vi "hdt_main_averageChannels.vi"(8 "outSteamSelect":u8(ring) items=["PID/ORT", "SICM"], 10 "hdt.p.averageEnabled":bool=TRUE, 11 "enableOutput":bool) -> (0 "debugStream":T1)   [LabVIEW 2016]
uses:
  <vilib>/rvi/Emulation/niFpgaEmulationIsFPGAContextNoSignature.vi
  <vilib>/rvi/Emulation/niFpgaSctlEmulationGetInTimedLoop.vi
  <vilib>/rvi/errors/niFpgaSetErrorForExecOnDevCompSimple.vi
  <vilib>/rvi/eio/common/nirviEmuReportErrorAndStop.vi
  <vilib>/rvi/DataTransferAndStorage/Container/Common/niFpgaContainerGetUniqueNameForEmu.vi
  <vilib>/rvi/FIFO/Fifo_Resource/nirvififoEmulationSetSize.vi
  <vilib>/rvi/FIFO/Fifo_Resource/nirviFifoEmulationQueueMgr.vi
  <instcachedir>/0/nirviFifoEmulationQueueMgr_E5CAEC123FF24DC58D834DCA3CDAA9B5.lvgen/nirviFifoEmulationQueueMgr_E5CAEC123FF24DC58D834DCA3CDAA9B5_010.vi
  <vilib>/Utility/error.llb/Clear Errors.vi
  <vilib>/rvi/FIFO/Fifo_Resource/nirvififoEmulationCreateLock.vi
  <vilib>/rvi/Emulation/niFpgaProcessEmulError.vi
  <vilib>/rvi/FIFO/Fifo_Resource/nirvififoEmulationObtainLock.vi
  <vilib>/rvi/FIFO/Fifo_Resource/nirvififoEmulationReleaseLock.vi
  <vilib>/rvi/occurrence/nirviWaitOnOccurrenceBase.vi
  <vilib>/rvi/errors/nirviReportUnexpectedCaseInternalError.vi
  <vilib>/rvi/errors/nirviReportUnexpectedCaseInternalError (U32).vi
  <instcachedir>/0/nirviFifoEmulationQueueMgr_E5CAEC123FF24DC58D834DCA3CDAA9B5.lvgen/nirviFifoEmulationQueueMgr_E5CAEC123FF24DC58D834DCA3CDAA9B5_009.vi
  <vilib>/rvi/FIFO/Fifo_Resource/nirvififoEmulationDetermineInputValidOut.vi
  <vilib>/rvi/DataTransferAndStorage/Container/XNode/niFpgaContainer.xnode
  <vilib>/rvi/FIFO/Fifo_Resource/nirvififoEmulationRead.vi
  <vilib>/rvi/FXPMathLib/FxpInterpret/XNode/nifxpmath_Interpret.xnode
  <vilib>/rvi/FIFO/Fifo_Resource/nirvififoEmulationWrite.vi
  <vilib>/eio/EIONode/EIONode.xnode
  <vilib>/rvi/eio/common/nirviEmuTemplateMethod_errors.vi
  <vilib>/rvi/DataTransferAndStorage/Register/Emulation/niFpgaRegisterEmulation.vi
types:
  T1 = cluster{"ch2":fxp<+/-,22,1>, "ch3":fxp<+/-,22,1>}
  T2 = cluster{"Element":fxp<+/-,22,1>, "Element":fxp<+/-,22,1>}
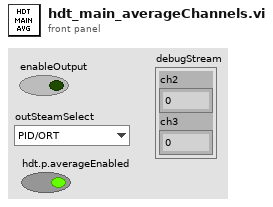
[diagram p1: front panel]
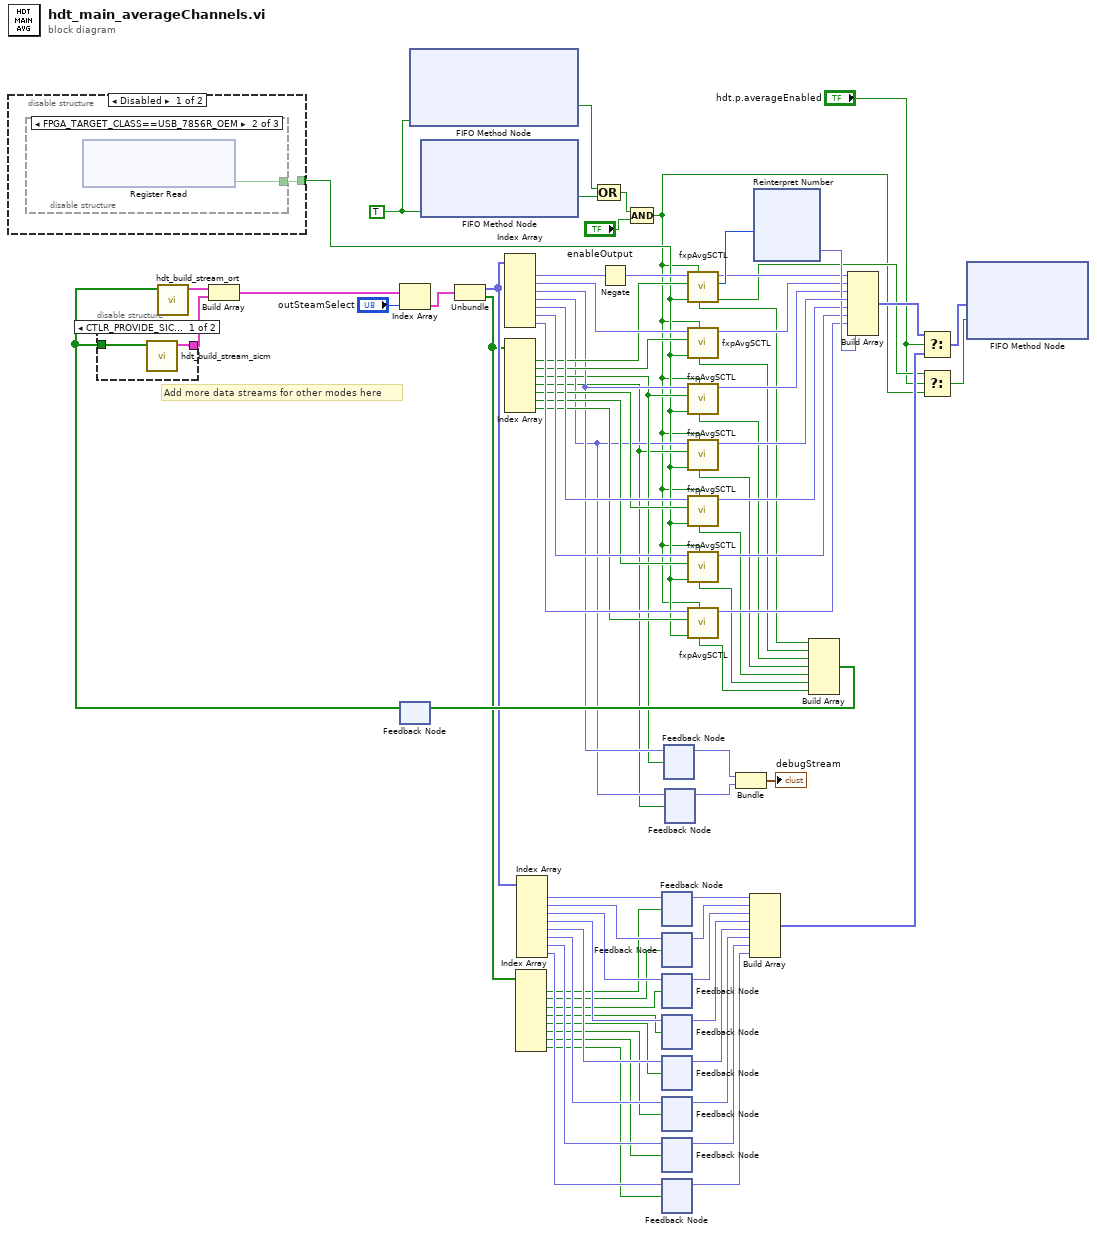
[diagram p0: block diagram]
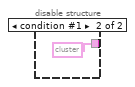
[diagram p2: hidden frame]
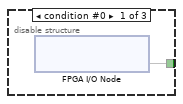
[diagram p3: hidden frame]
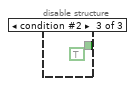
[diagram p4: hidden frame]
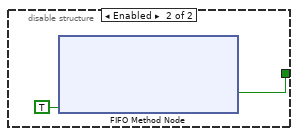
[diagram p5: hidden frame]
diagram:
  w43 = TRUE ("Ready for Output")
  # "Add more data streams for other modes here"
  n1 = disable-structure shown="Disabled" {
    disable-tunnel: [w81 w86] -> w34
    frame Disabled {
      n2 = disable-structure shown="FPGA_TARGET_CLASS==USB_7856R_OEM" {
        disable-tunnel: [w82 w83 TRUE ("outputEnable")] -> w81
        frame condition #0 {
          n3 = xnode "FPGA I/O Node"() -> ("outputEnable"=w82)  [unwired: 1 in, 1 out]
        }
        frame condition #1 (active) {
          n4 = xnode ("Register Read")() -> ("Data"=w83:bool)  [unwired: 1 in, 1 out]
        }
        frame condition #2 {
        }
      }
    }
    frame Enabled {
      n5 = xnode ("FIFO Method Node")("Ready for Output"=TRUE) -> ("Output Valid"=w86:bool)  [unwired: 1 in, 2 out]
    }
  }
  n6 = feedback #1() -> (w52:bool[])  [unwired: 1 in]
  n7 = disable-structure shown="CTLR_PROVIDE_SICM==1" {
    disable-tunnel: w52 -> [w88 _]
    disable-tunnel: [w87 cluster{fxp<+/-,22,1>[], bool[]} {[0.0, 0.0, 0.0, 0.0, 0.0, 0.0, 0.0], [FALSE, FALSE, FALSE, FALSE, FALSE, FALSE, FALSE]} ("dataStream")] -> w51
    frame condition #0 (active) {
      n8 = call "hdt_build_stream_sicm.vi"("readyForOutput"=w88) -> ("dataStream"=w87:cluster{fxp<+/-,22,1>[], bool[]})  [unwired: 10 in]
    }
    frame condition #1 {
    }
  }
  n9 = call "hdt_build_stream_ort.vi"("readyForOutput"=w52) -> ("dataStream"=w70:cluster{fxp<+/-,22,1>[], bool[]})  [unwired: 10 in]
  n10 = Build Array(w70, w51) -> (w69:cluster{fxp<+/-,22,1>[], bool[]}[])
  n11 = Index Array(array=w69, index="outSteamSelect") -> (element=w67:cluster{fxp<+/-,22,1>[], bool[]})
  n12 = xnode ("FIFO Method Node")("Ready for Output"=w43) -> ("Output Valid"=w42:bool)  [unwired: 1 in, 2 out]
  n13 = xnode ("FIFO Method Node")("Ready for Output"=w43) -> ("Output Valid"=w46:bool)  [unwired: 1 in, 2 out]
  n14 = Unbundle(w67) -> (w33:fxp<+/-,22,1>[], w24:bool[])
  n15 = Index Array(array=w33) -> (element #1=w66:fxp<+/-,22,1>, element #2=w65:fxp<+/-,22,1>, element #3=w41:fxp<+/-,22,1>, element #4=w39:fxp<+/-,22,1>, element #5=w64:fxp<+/-,22,1>, element #6=w63:fxp<+/-,22,1>, element #7=w62:fxp<+/-,22,1>)  [unwired: 7 in]
  n16 = Index Array(array=w24) -> (element #1=w53:bool, element #2=w50:bool, element #3=w40:bool, element #4=w38:bool, element #5=w49:bool, element #6=w48:bool, element #7=w47:bool)  [unwired: 7 in]
  n17 = Index Array(array=w24) -> (element #1=w3:bool, element #2=w23:bool, element #3=w22:bool, element #4=w21:bool, element #5=w20:bool, element #6=w19:bool, element #7=w18:bool, element #8=w17:bool)  [unwired: 8 in]
  n18 = Index Array(array=w33) -> (element #1=w32:fxp<+/-,22,1>, element #2=w31:fxp<+/-,22,1>, element #3=w30:fxp<+/-,22,1>, element #4=w29:fxp<+/-,22,1>, element #5=w28:fxp<+/-,22,1>, element #6=w27:fxp<+/-,22,1>, element #7=w26:fxp<+/-,22,1>, element #8=w25:fxp<+/-,22,1>)  [unwired: 8 in]
  n19 = Compound Arithmetic op=OR(w42, w46) -> (w44:bool)
  n20 = Negate(x=w66) -> (-x=w80:fxp<+/-,23,2>)
  n21 = Compound Arithmetic op=AND(w44, "enableOutput") -> (w1:bool)
  n22 = feedback-in #2(w32, w3) -> ()
  n23 = feedback #2() -> (w16:fxp<+/-,22,1>)  [unwired: 1 in]
  n24 = feedback #3() -> (w15:fxp<+/-,22,1>)  [unwired: 1 in]
  n25 = feedback-in #3(w31, w23) -> ()
  n26 = feedback #4() -> (w9:fxp<+/-,22,1>)  [unwired: 1 in]
  n27 = feedback-in #4(w30, w22) -> ()
  n28 = feedback #5() -> (w10:fxp<+/-,22,1>)  [unwired: 1 in]
  n29 = feedback-in #5(w29, w21) -> ()
  n30 = feedback #6() -> (w11:fxp<+/-,22,1>)  [unwired: 1 in]
  n31 = feedback-in #6(w28, w20) -> ()
  n32 = feedback #7() -> (w12:fxp<+/-,22,1>)  [unwired: 1 in]
  n33 = feedback-in #7(w27, w19) -> ()
  n34 = feedback #8() -> (w13:fxp<+/-,22,1>)  [unwired: 1 in]
  n35 = feedback-in #8(w26, w18) -> ()
  n36 = feedback #9() -> (w14:fxp<+/-,22,1>)  [unwired: 1 in]
  n37 = feedback-in #9(w25, w17) -> ()
  n38 = feedback-in #10(w41, w40) -> ()
  n39 = feedback #10() -> (w37:fxp<+/-,22,1>)  [unwired: 1 in]
  n40 = feedback #11() -> (w36:fxp<+/-,22,1>)  [unwired: 1 in]
  n41 = feedback-in #11(w39, w38) -> ()
  n42 = call "fxpAvgSCTL.vi"("reset"=w1, "clear"=w34, "inputValid"=w53, "input"=w80) -> ("outputValid"=w5:bool, "noAvg"=w77:u16, "average"=w71:fxp<+/-,22,1>, "readyForInput"=w61:bool)  [unwired: 4 in]
  n43 = call "fxpAvgSCTL.vi"("reset"=w1, "clear"=w34, "inputValid"=w50, "input"=w65) -> ("average"=w72:fxp<+/-,22,1>, "readyForInput"=w60:bool)  [unwired: 4 in, 2 out]
  n44 = call "fxpAvgSCTL.vi"("reset"=w1, "clear"=w34, "inputValid"=w40, "input"=w41) -> ("average"=w73:fxp<+/-,22,1>, "readyForInput"=w59:bool)  [unwired: 4 in, 2 out]
  n45 = call "fxpAvgSCTL.vi"("reset"=w1, "clear"=w34, "inputValid"=w38, "input"=w39) -> ("average"=w79:fxp<+/-,22,1>, "readyForInput"=w58:bool)  [unwired: 4 in, 2 out]
  n46 = call "fxpAvgSCTL.vi"("reset"=w1, "clear"=w34, "inputValid"=w49, "input"=w64) -> ("average"=w74:fxp<+/-,22,1>, "readyForInput"=w57:bool)  [unwired: 4 in, 2 out]
  n47 = call "fxpAvgSCTL.vi"("reset"=w1, "clear"=w34, "inputValid"=w48, "input"=w63) -> ("average"=w75:fxp<+/-,22,1>, "readyForInput"=w56:bool)  [unwired: 4 in, 2 out]
  n48 = call "fxpAvgSCTL.vi"("reset"=w1, "clear"=w34, "inputValid"=w47, "input"=w62) -> ("average"=w76:fxp<+/-,22,1>, "readyForInput"=w55:bool)  [unwired: 4 in, 2 out]
  n49 = Bundle("Element"=w37, "Element"=w36) -> (→"debugStream":T2)  [unwired: 1 in]
  n50 = Build Array(w16, w15, w9, w10, w11, w12, w13, w14) -> (w7:fxp<+/-,22,1>[])
  n51 = xnode "Reinterpret Number"("x"=w77) -> ("y"=w78:fxp<+,16,1>)
  n52 = Build Array(w61, w60, w59, w58, w57, w56, w55) -> (w54:bool[])
  n53 = feedback-in #1(w54) -> ()
  n54 = Build Array(w71, w72, w73, w79, w74, w75, w76, w78) -> (w6:fxp<+/-,23,2>[])
  n55 = Select(t=w6, s="hdt.p.averageEnabled", f=w7) -> (s? t:f=w8:fxp<+/-,23,2>[])
  n56 = Select(t=w5, s="hdt.p.averageEnabled", f=w1) -> (s? t:f=w4:bool)
  n57 = xnode ("FIFO Method Node")("Element"=w8, "Input Valid"=w4) -> ()  [unwired: 1 in, 2 out]
